vi "GetCircleResultNames.vi"(7 "ProjectName":string="Prj", 10 "Analysis_Circle_Parameter":T1={"ROI Descriptor"={"Global Rectangle"=[], "Contours"=[]}, "Options"={"Search  Direction"=0, "Edge Options"={"Edge Polarity"=0, "Kernel Size"=3, "Width"=3, "Minimum Edge Strength"=10.0, "Interpolation Type"=enum."Bilinear Fixed", "Data Processing Method"=enum."Average"}, "Show Search Area"=FALSE, "Show Search Lines"=FALSE, "Show Edges Found"=FALSE, "Show Result"=TRUE, "Search Area Color"=65280, "Search Lines Color"=255, "Edge Locations Color"=16776960, "Result Color"=16711680, "Overlay Group Name"=""}, "Circle Fit Options"={"Process"=enum."Get First Edge", "Step Size"=3.0, "Max Pixel Radius"=3}} {"Options"."Search  Direction" items=["Outside to Inside", "Inside to Outside"]; "Options"."Edge Options"."Edge Polarity" items=["All Edges", "Rising Edges", "Falling Edges"]; "Options"."Edge Options"."Minimum Edge Strength" format="%.2f"; "Options"."Edge Options"."Width" step=2; "Options"."Edge Options"."Kernel Size" step=2}, 11 "ROI_Name":string="ROI1") -> (3 "ResultNames":string[](array[string]))   [LabVIEW 2019]
uses:
  Controls/Circle/Analysis_Circle_Result.ctl
  Controls/Circle/Analysis_Circle_Parameter.ctl
  <vilib>/vision/Measure.llb/Edge Options.ctl
  <vilib>/vision/Measure.llb/Edge Polarity.ctl
panel:
  in  "Analysis_Clamp_Result":T4 {"Fitted Circle"."Average SNR (dB)" format="%.2f"; "Fitted Circle"."Average Strength" format="%.2f"; "Fitted Circle"."Roundness (Real-World)" format="%.2f"; "Fitted Circle"."Radius (Real-World)" format="%.2f"; "Fitted Circle"."Center (Real-World)"."Y" format="%.2f"; "Fitted Circle"."Center (Real-World)"."X" format="%.2f"; "Fitted Circle"."Radius (Pixels)" format="%.2f"; "Fitted Circle"."Center (Pixels)"."Y" format="%.2f"; "Fitted Circle"."Center (Pixels)"."X" format="%.2f"}
  out "error out":errorcluster
  in  "error in (no error)":errorcluster
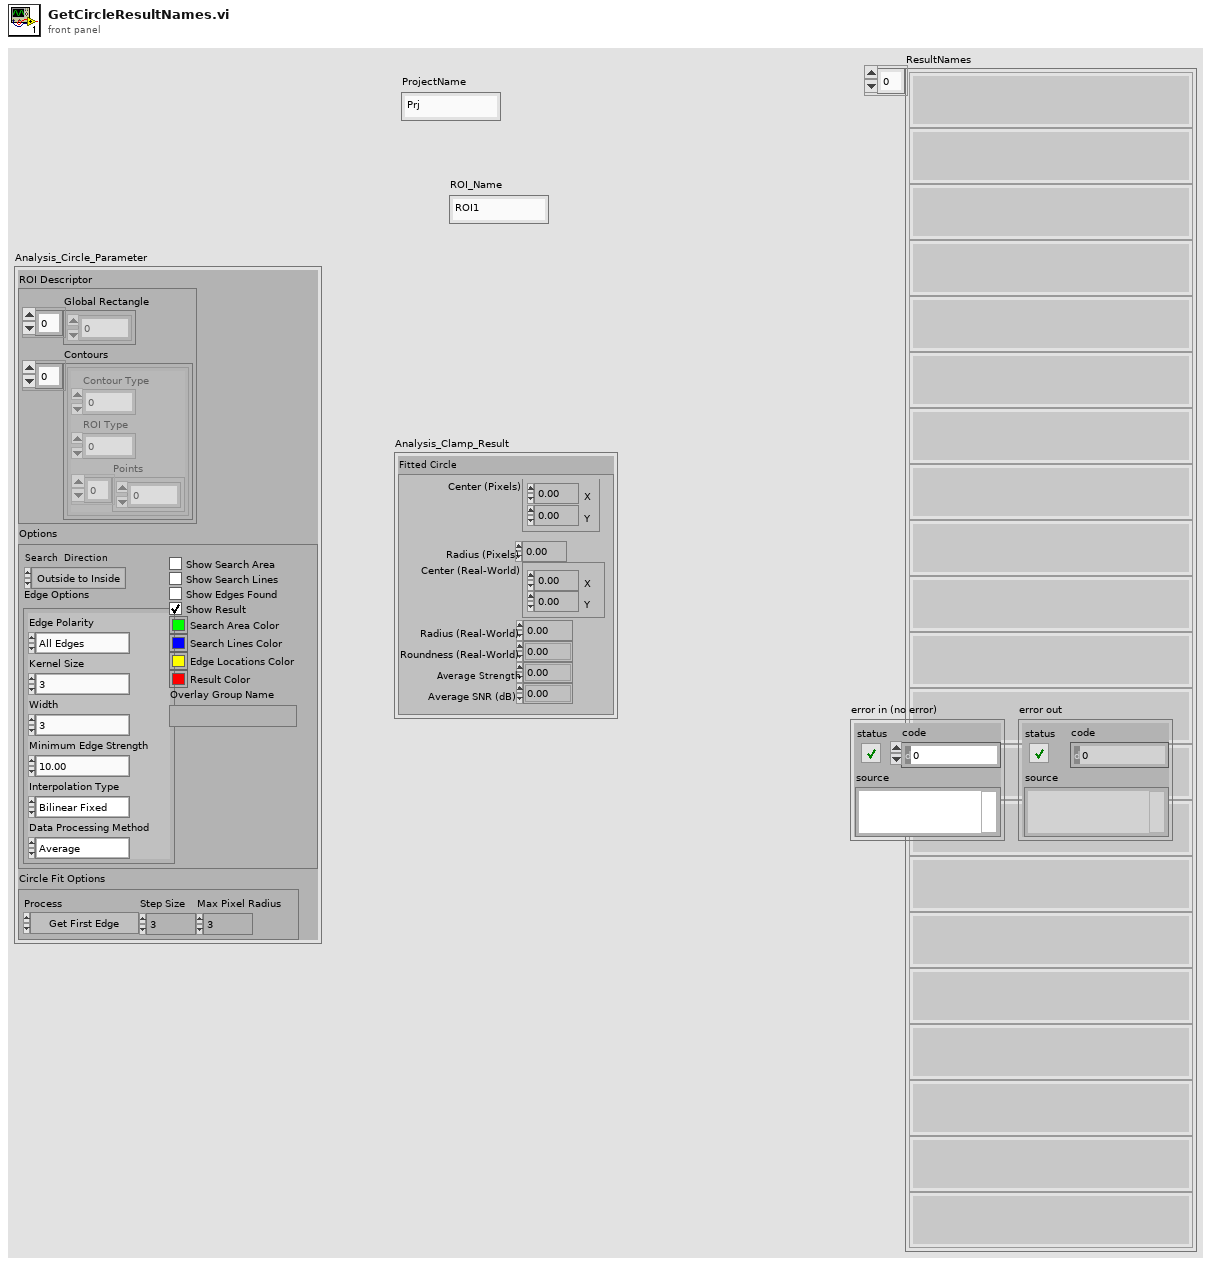
[diagram p1: front panel]
types:
  T1 = typedef "Analysis_Circle_Parameter.ctl" = cluster{"ROI Descriptor":cluster{"Global Rectangle":i32[], "Contours":cluster{"Contour Type":u32, "ROI Type":u32, "Points":i32[]}[]}, "Options":cluster{"Search  Direction":u32, "Edge Options":T2, "Show Search Area":bool, "Show Search Lines":bool, "Show Edges Found":bool, "Show Result":bool, "Search Area Color":u32, "Search Lines Color":u32, "Edge Locations Color":u32, "Result Color":u32, "Overlay Group Name":string}, "Circle Fit Options":cluster{"Process":enum16{"Get First Edge", "Get First + Last Edge", "Get All Edges", "Get Best Edge"}, "Step Size":dbl, "Max Pixel Radius":i32}}
  T2 = typedef "Edge Options.ctl" = cluster{"Edge Polarity":T3, "Kernel Size":u32, "Width":u32, "Minimum Edge Strength":sgl, "Interpolation Type":enum32{"Zero Order", "Bilinear", "Quadratic", "Cubic", "Bilinear Fixed"}, "Data Processing Method":enum32{"Average", "Median"}}
  T3 = typedef "Edge Polarity.ctl" = u32
  T4 = typedef "Analysis_Circle_Result.ctl" = cluster{"Fitted Circle":cluster{"Center (Pixels)":cluster{"X":sgl, "Y":sgl}, "Radius (Pixels)":dbl, "Center (Real-World)":cluster{"X":sgl, "Y":sgl}, "Radius (Real-World)":dbl, "Roundness (Real-World)":dbl, "Average Strength":dbl, "Average SNR (dB)":dbl}}
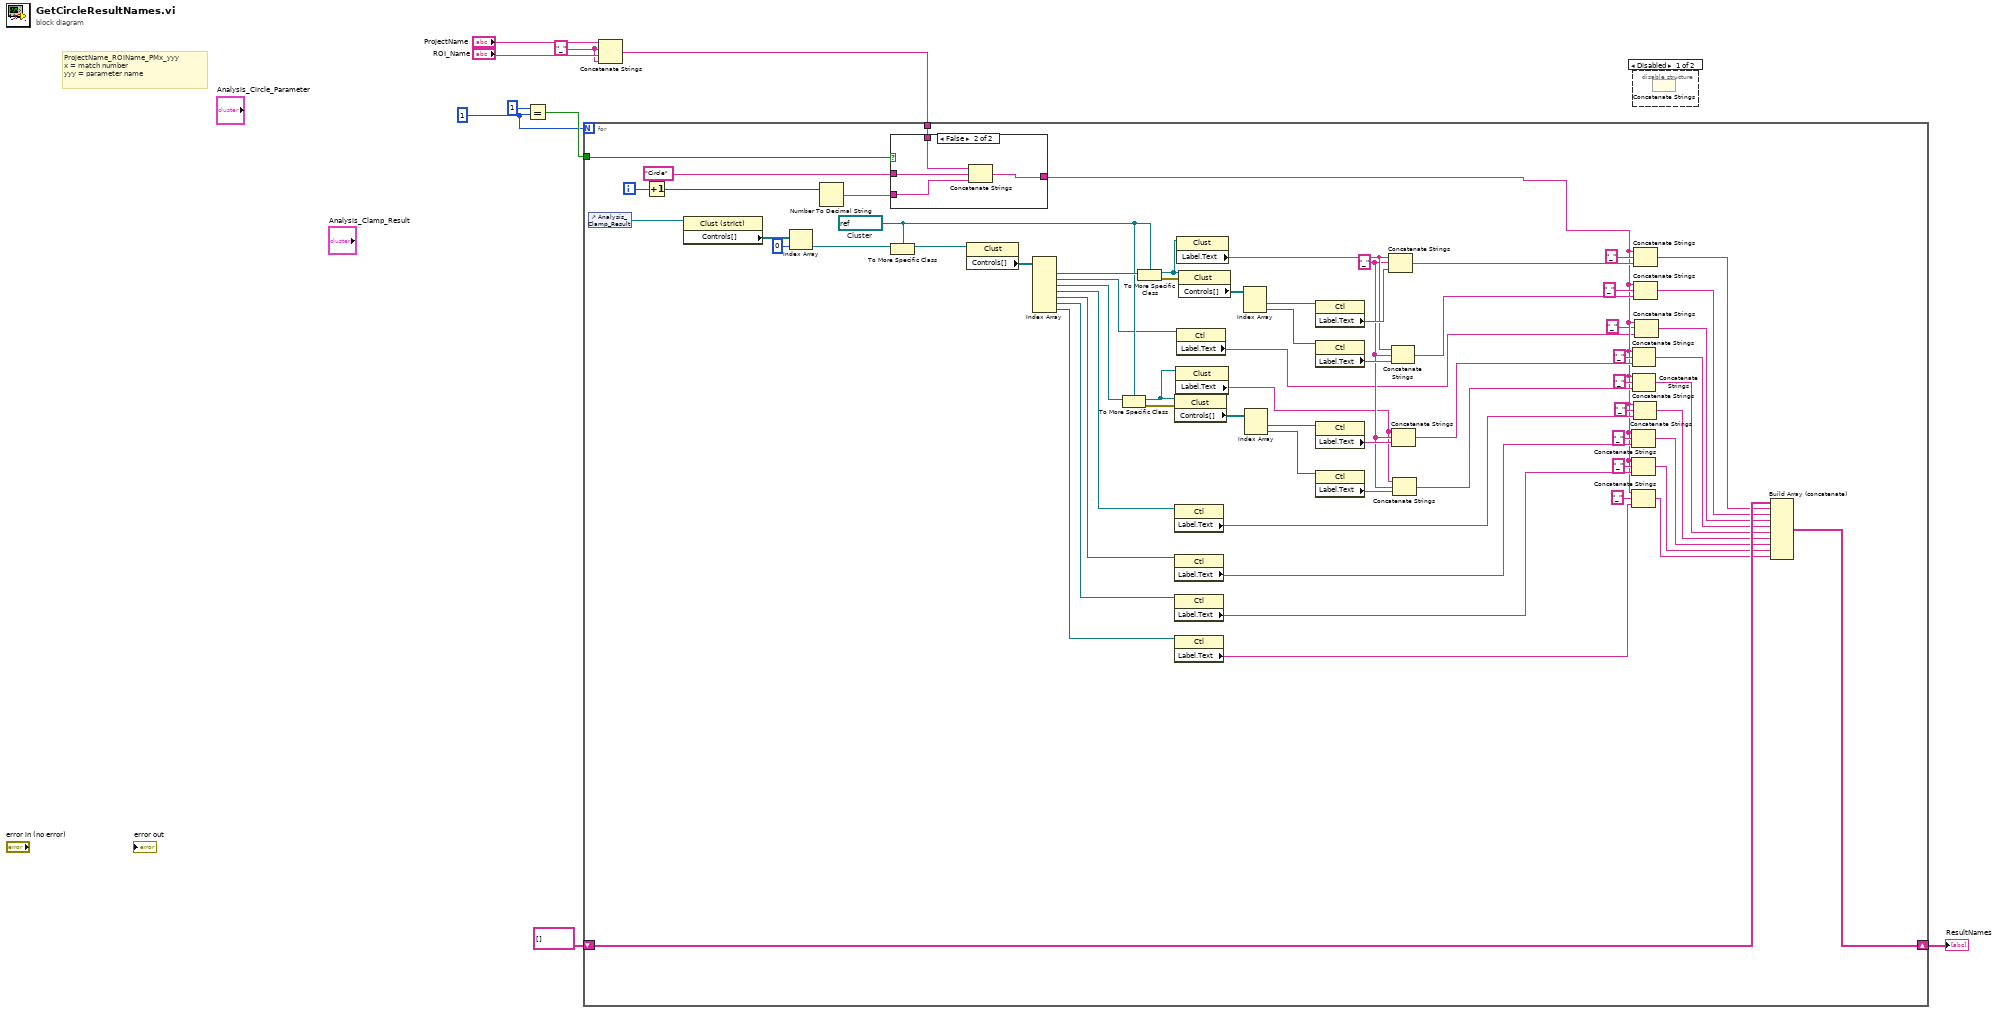
[diagram p0: block diagram]
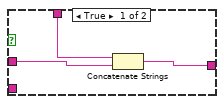
[diagram p3: hidden frame]
diagram:
  w1 = 1
  w7 = "_" ("string")
  # "ProjectName_ROIName_PMx_yyy\nx = match number\nyyy = parameter name"
  n1 = Equal?(x=1, y=w1) -> (x = y?=w3:bool)
  n2 = Concatenate Strings("ProjectName", w7, "ROI_Name", w7) -> (w6:string)
  n3 = for {
    N: w1 -> [_]
    tunnel: w6 -> [w74]
    shift-right: [w69] -> w4
    shift-left: string[] [] -> [w70]
    tunnel: w3 -> [w75]
    i -> [w71]
    w41 = "_"
    w48 = refnum<vi> refnum  # Cluster
    n4 = control-ref of="Analysis_Clamp_Result"() -> (w61:refnum<vi>)
    n5 = Increment(x=w71) -> (x+1=w76:i32)
    n6 = property class="Clust (strict)"(reference=w61) -> ("Controls[]"=w60:refnum<vi>[])  [unwired: 1 in, 2 out]
    n7 = Index Array(array=w60, index=0) -> (element=w59:refnum<vi>)
    n8 = Number To Decimal String(number=w76) -> (decimal integer string=w73:string)  [unwired: 1 in]
    n9 = case shown="False" w75 {
      tunnel: w74 -> [w79 w83]
      tunnel: w73 -> [_ w81]
      tunnel: [w78 w82] -> w15
      tunnel: "Circle" ("string") -> [w77 w80]
      frame True {
        n10 = Concatenate Strings(w79, w77) -> (w78:string)
      }
      frame False {
        n11 = Concatenate Strings(w83, w80, w81) -> (w82:string)
      }
    }
    n12 = To More Specific Class(target class=w48, reference=w59) -> (specific class reference=w58:refnum<vi>)  [unwired: 1 in, 1 out]
    n13 = property class="Clust"(reference=w58) -> ("Controls[]"=w57:refnum<vi>[])  [unwired: 1 in, 2 out]
    n14 = Index Array(array=w57) -> (element #1=w56:refnum<vi>, element #2=w37:refnum<vi>, element #3=w38:refnum<vi>, element #4=w36:refnum<vi>, element #5=w35:refnum<vi>, element #6=w34:refnum<vi>, element #7=w33:refnum<vi>)  [unwired: 7 in]
    n15 = To More Specific Class(target class=w48, reference=w38) -> (specific class reference=w11:refnum<vi>, error out=w47:errorcluster)  [unwired: 1 in]
    n16 = To More Specific Class(target class=w48, reference=w56) -> (specific class reference=w51:refnum<vi>, error out=w55:errorcluster)  [unwired: 1 in]
    n17 = property class="Clust"(reference=w11, error in=w47) -> ("Controls[]"=w46:refnum<vi>[])  [unwired: 2 out]
    n18 = property class="Ctl"(reference=w36) -> ("Label.Text"=w22:string)  [unwired: 1 in, 2 out]
    n19 = property class="Ctl"(reference=w35) -> ("Label.Text"=w21:string)  [unwired: 1 in, 2 out]
    n20 = property class="Ctl"(reference=w34) -> ("Label.Text"=w20:string)  [unwired: 1 in, 2 out]
    n21 = property class="Ctl"(reference=w33) -> ("Label.Text"=w17:string)  [unwired: 1 in, 2 out]
    n22 = property class="Clust"(reference=w11) -> ("Label.Text"=w10:string)  [unwired: 1 in, 2 out]
    n23 = property class="Clust"(reference=w51) -> ("Label.Text"=w42:string)  [unwired: 1 in, 2 out]
    n24 = property class="Ctl"(reference=w37) -> ("Label.Text"=w13:string)  [unwired: 1 in, 2 out]
    n25 = property class="Clust"(reference=w51, error in=w55) -> ("Controls[]"=w54:refnum<vi>[])  [unwired: 2 out]
    n26 = Index Array(array=w54) -> (element #1=w53:refnum<vi>, element #2=w52:refnum<vi>)  [unwired: 2 in]
    n27 = Index Array(array=w46) -> (element #1=w45:refnum<vi>, element #2=w44:refnum<vi>)  [unwired: 2 in]
    n28 = property class="Ctl"(reference=w53) -> ("Label.Text"=w50:string)  [unwired: 1 in, 2 out]
    n29 = property class="Ctl"(reference=w52) -> ("Label.Text"=w49:string)  [unwired: 1 in, 2 out]
    n30 = property class="Ctl"(reference=w45) -> ("Label.Text"=w43:string)  [unwired: 1 in, 2 out]
    n31 = property class="Ctl"(reference=w44) -> ("Label.Text"=w40:string)  [unwired: 1 in, 2 out]
    n32 = Concatenate Strings(w42, w41, w50) -> (w26:string)
    n33 = Concatenate Strings(w42, w41, w49) -> (w25:string)
    n34 = Concatenate Strings(w10, w41, w43) -> (w24:string)
    n35 = Concatenate Strings(w10, w41, w40) -> (w23:string)
    n36 = Concatenate Strings(w15, "_" ("string"), w21) -> (w63:string)
    n37 = Concatenate Strings(w15, "_" ("string"), w20) -> (w62:string)
    n38 = Concatenate Strings(w15, "_" ("string"), w17) -> (w16:string)
    n39 = Concatenate Strings(w15, "_" ("string"), w24) -> (w66:string)
    n40 = Concatenate Strings(w15, "_" ("string"), w23) -> (w65:string)
    n41 = Concatenate Strings(w15, "_" ("string"), w22) -> (w64:string)
    n42 = Concatenate Strings(w15, "_" ("string"), w26) -> (w68:string)
    n43 = Concatenate Strings(w15, "_" ("string"), w25) -> (w67:string)
    n44 = Concatenate Strings(w15, "_", w13) -> (w12:string)
    n45 = Build Array (concatenate)(w70, w68, w67, w12, w66, w65, w64, w63, w62, w16) -> (w69:string[])
  }
  "ResultNames" <- w4
  n46 = disable-structure shown="Disabled" {
    frame Disabled {
      n47 = Concatenate Strings() -> ()  [unwired: 2 in, 1 out]
    }
    frame Enabled {
    }
  }
